vi "Do Add To Selection.vi"(8 "error in (no error)":errorcluster, 10 "add_to_selection Argument":T2, 11 "Data Cluster in":T1) -> (0 "error out":errorcluster, 3 "Data Cluster out":T1)   [LabVIEW 2025, in "Scripting Server.lvlib"]
uses:
  Scripting Server.lvlib
  add_to_selection Argument--cluster.ctl
  add_to_selection (Reply Payload)--cluster.ctl
  Module Data--cluster.ctl
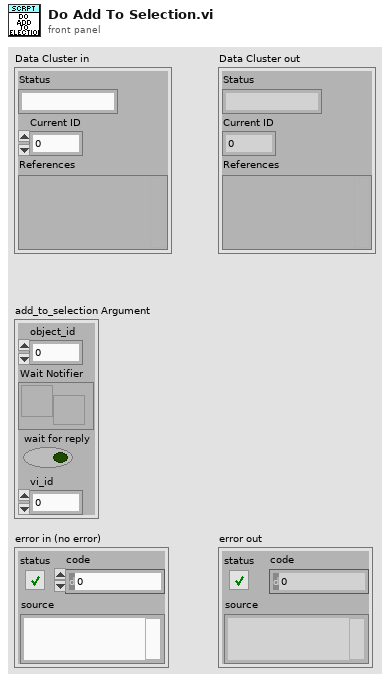
[diagram p1: front panel]
types:
  T1 = typedef "Scripting Server.lvlib/Module Data--cluster.ctl" = cluster{"Status":string, "Current ID":i32, "References":variant}
  T2 = typedef "Scripting Server.lvlib/add_to_selection Argument--cluster.ctl" = cluster{"object_id":i32, "Wait Notifier":refnum<notifier>, "wait for reply":bool, "vi_id":i32}
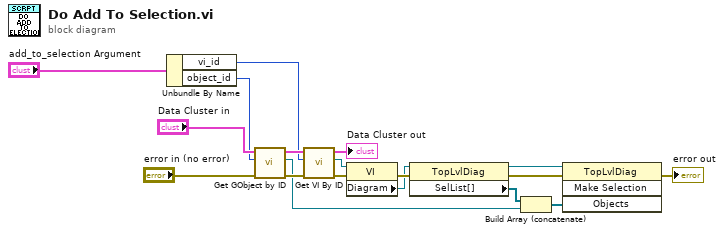
[diagram p0: block diagram]
diagram:
  n1 = Unbundle By Name("add_to_selection Argument") -> ("vi_id"=w1:i32, "object_id"=w3:i32)
  n2 = call "Get GObject by ID.vi"("error in (no error)"="error in (no error)", "ID"=w3, "Data Cluster in"="Data Cluster in") -> ("error out"=w6:errorcluster, "gobject"=w2:refnum<vi>, "Data Cluster out"=w4:T1)  [unwired: 6 in]
  n3 = call "Get VI By ID.vi"("error in (no error)"=w6, "ID"=w1, "Data Cluster in"=w4) -> ("error out"=w16:errorcluster, "VI Reference"=w14:refnum<vi>, "Data Cluster out"=→"Data Cluster out":T1)  [unwired: 6 in]
  n4 = property class="VI"(reference=w14, error in=w16) -> (error out=w12:errorcluster, "Diagram"=w10:refnum<vi>)  [unwired: 1 out]
  n5 = property class="TopLvlDiag"(reference=w10, error in=w12) -> (reference out=w9:refnum<vi>, error out=w11:errorcluster, "SelList[]"=w8:refnum<vi>[])
  n6 = Build Array (concatenate)(w8, w2) -> (w7:refnum<vi>[])
  n7 = invoke class="TopLvlDiag" method="Make Selection"(reference=w9, error in=w11, "Objects"=w7) -> (error out=→"error out":errorcluster)  [unwired: 1 in, 3 out]
